vi "InitializeTestDatabase.vi"(8 "error in (no error)":errorcluster, 11 "VariableManager in":refnum<class "VariableManager.lvclass">) -> (0 "error out":errorcluster, 3 "VariableManager out":refnum<class "VariableManager.lvclass">)   [LabVIEW 2013, in "VariableManager.lvclass"]
doc: "Initialize variable manager database for testing."
uses:
  VariableManager.lvclass
  Variable/Variable.lvclass
  SequenceIndex/SequenceIndex.lvclass
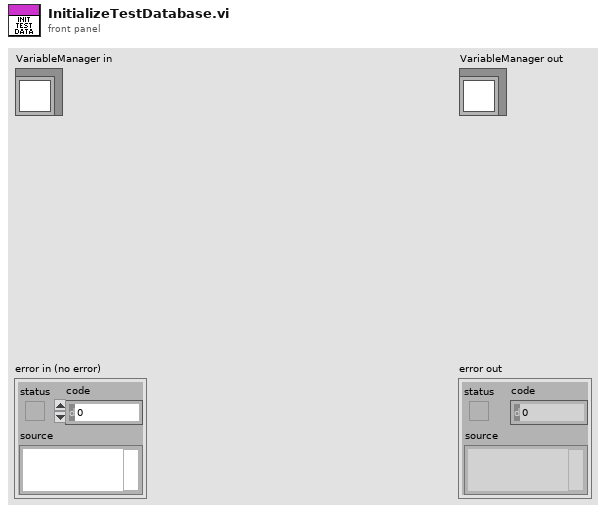
[diagram p1: front panel]
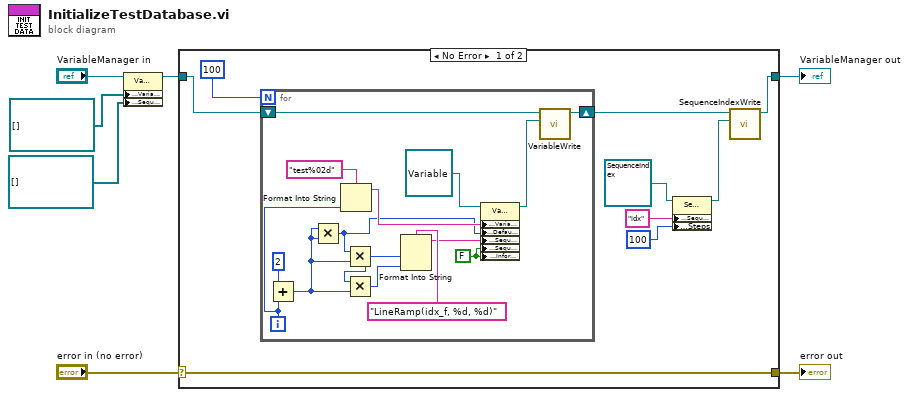
[diagram p0: block diagram]
diagram:
  n1 = property class="VariableManager.lvclass"(reference="VariableManager in", "Accessors:Variables"=refnum<class "Variable.lvclass">[] [] ("Variables"), "Accessors:SequenceIndices"=refnum<class "SequenceIndex.lvclass">[] [] ("SequenceIndices")) -> (reference out=w3:refnum<class "VariableManager.lvclass">)  [unwired: 1 in, 1 out]
  n2 = case shown="No Error" "error in (no error)" {
    selector: "error in (no error)" -> [w16 w33]
    tunnel: [w16 w33] -> w6
    tunnel: [w10 w32] -> w5
    tunnel: w3 -> [w14 w32]
    frame No Error {
      n3 = for {
        N: 100 -> [_]
        shift-right: [w27] -> w11
        shift-left: w14 -> [w17]
        i -> [w20]
        w26 = FALSE ("Sequence")
        n4 = Add(x=2, y=w20) -> (x+y=w18:i32)
        n5 = Multiply(x=w18, y=w18) -> (x*y=w23:i32)
        n6 = Format Into String(format string="test%02d", w20) -> (resulting string=w24:string)  [unwired: 2 in, 1 out]
        n7 = Multiply(x=w23, y=w18) -> (x*y=w22:i32)
        n8 = Multiply(x=w22, y=w18) -> (x*y=w21:i32)
        n9 = Format Into String(format string="LineRamp(idx_f, %d, %d)", w22, w21) -> (resulting string=w28:string)  [unwired: 2 in, 1 out]
        n10 = property class="Variable.lvclass"(reference=refnum<class "Variable.lvclass"> refnum ("Variable.lvclass"), "Accessors:VariableName"=w24, "Accessors:DefaultValue"=w23, "Accessors:SequenceFunction"=w28, "Accessors:Sequence"=w26, "Accessors:InformIgor"=w26) -> (reference out=w31:refnum<class "Variable.lvclass">)  [unwired: 1 in, 1 out]
        n11 = call-dynamic "VariableWrite.vi"("Variable"=w31, "VariablesManager in"=w17) -> ("VariablesManager out"=w27:refnum<class "VariableManager.lvclass">)  [unwired: 8 in, 1 out]
      }
      n12 = property class="SequenceIndex.lvclass"(reference=refnum<class "SequenceIndex.lvclass"> refnum ("SequenceIndex.lvclass"), "Accessors:SequenceIndexName"="idx", "Accessors:Steps"=u32 100 ("Steps")) -> (reference out=w12:refnum<class "SequenceIndex.lvclass">)  [unwired: 1 in, 1 out]
      n13 = call-dynamic "SequenceIndexWrite.vi"("SequenceIndex"=w12, "VariableManager in"=w11) -> ("VariableManager out"=w10:refnum<class "VariableManager.lvclass">)  [unwired: 8 in, 1 out]
    }
    frame Error {
    }
  }
  "error out" <- w6
  "VariableManager out" <- w5
